vi "TCP test.vi"() -> ()   [LabVIEW 2010]
panel:
  out "String":string
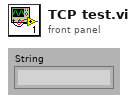
[diagram p1: front panel]
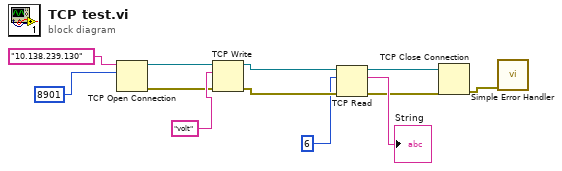
[diagram p0: block diagram]
diagram:
  n1 = TCP Open Connection(address="10.138.239.130", remote port or service name=u16 8901) -> (connection ID=w10:refnum<k5>, error out=w5:errorcluster)  [unwired: 3 in]
  n2 = TCP Write(connection ID=w10, data in="volt", error in (no error)=w5) -> (connection ID out=w9:refnum<k5>, error out=w4:errorcluster)  [unwired: 1 in, 1 out]
  n3 = TCP Read(connection ID=w9, bytes to read=6, error in (no error)=w4) -> (connection ID out=w8:refnum<k5>, data out=→"String":string, error out=w3:errorcluster)  [unwired: 2 in]
  n4 = TCP Close Connection(connection ID=w8, error in (no error)=w3) -> (error out=w2:errorcluster)  [unwired: 1 in, 1 out]
  n5 = call <vilib>:"Simple Error Handler.vi"("error in (no error)"=w2) -> ()  [unwired: 4 in, 5 out]
